vi "Find One by ID.vi"(7 "Entity ID":T1, 8 "error in (no error)":errorcluster, 9 "Entity Definition":refnum<class "Type.lvclass">[](array[class]), 10 "Table Name":string, 11 "Database in":refnum<class "Database Platform.lvclass">) -> (0 "error out":errorcluster, 2 "Result Row":refnum<class "Result Row.lvclass">, 3 "Database out":refnum<class "Database Platform.lvclass">)   [LabVIEW 2020, in "Conditu2.lvlib" / "Database Platform.lvclass"]
uses:
  Database Platform.lvclass
  Columns/Type/Type.lvclass
  Result Row/Result Row.lvclass
  Entity ID.ctl
  Conditu2.lvlib
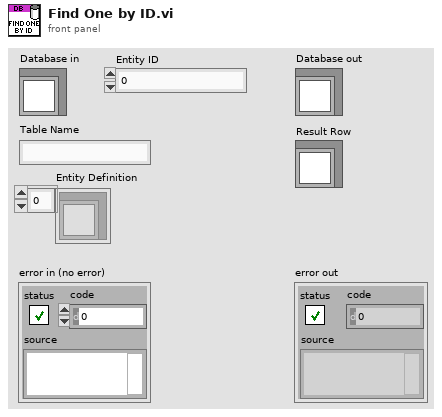
[diagram p1: front panel]
types:
  T1 = typedef "Conditu2.lvlib/Entity ID.ctl" = i64
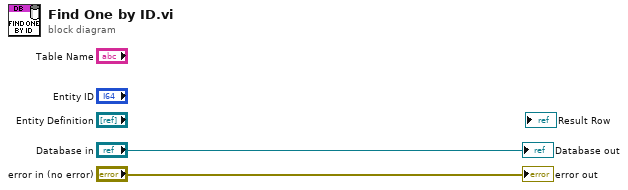
[diagram p0: block diagram]
diagram:
  "error out" <- "error in (no error)"
  "Database out" <- "Database in"
